vi "EnqueueMessage.vi"(8 "error in (no error)":errorcluster, 9 "Priority":u8, 10 "message":variant, 11 "queue in":refnum<data-value>) -> (0 "error out":errorcluster, 3 "queue out":refnum<data-value>)   [LabVIEW 2009, in "PriorityQueue.lvlib"]
uses:
  PriorityQueue.lvlib
  PriorityQueue/PriorityQueue.lvclass
  LLNode/LLNode.lvclass
  LinkedList/InsertSearch.ctl
  LLSearch/LLSearch.lvclass
  SearchPriority/SearchPriority.lvclass
  PriorityNode/PriorityNode.lvclass
  LinkedList/position.ctl
  LinkedList/LinkedList.lvclass
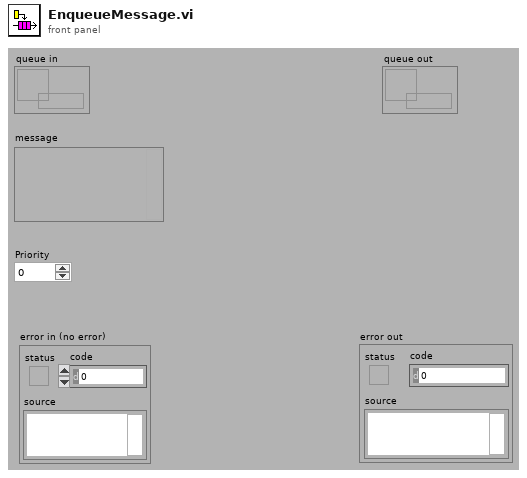
[diagram p1: front panel]
types:
  T1 = typedef "LinkedList.lvclass/InsertSearch.ctl" = cluster{"LLSearch in":refnum<class "LLSearch.lvclass">, "InsertIfEmpty":bool, "Insert After":bool, "InsertIfNotFound":bool}
  T2 = typedef "LinkedList.lvclass/position.ctl" = enum16{"Front", "Back", "Search"}
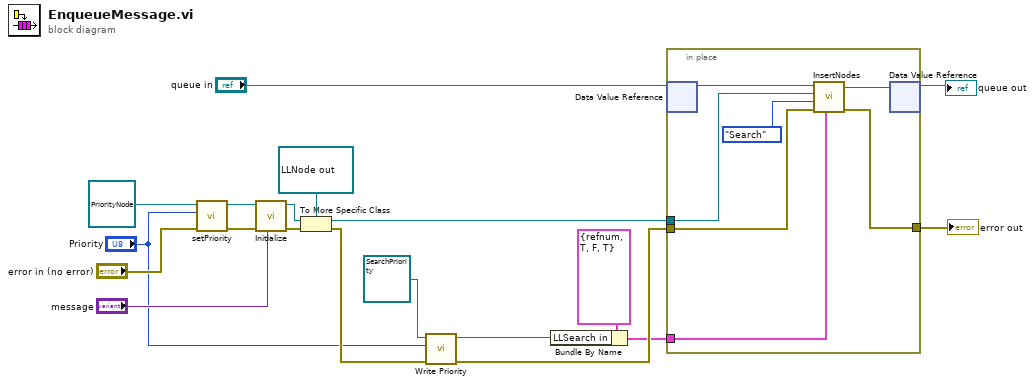
[diagram p0: block diagram]
diagram:
  n1 = call "setPriority.vi"("error in (no error)"="error in (no error)", "Priority"="Priority", "PriorityNode in"=refnum<class "PriorityNode.lvclass"> refnum ("PriorityNode.lvclass")) -> ("error out"=w2:errorcluster, "PriorityNode out"=w4:refnum<class "PriorityNode.lvclass">)  [unwired: 7 in]
  n2 = call-dynamic "Initialize.vi"("optional"="message", "error in (no error)"=w2, "PriorityNode data"=w4) -> ("error out"=w18:errorcluster, "Node out"=w17:refnum<data-value>)  [unwired: 7 in]
  n3 = To More Specific Class(target class=refnum<data-value> refnum ("ToInsert"), reference=w17, error in=w18) -> (specific class reference=w15:refnum<data-value>, error out=w13:errorcluster)
  n4 = call "Write Priority.vi"("error in (no error)"=w13, "Priority"="Priority", "SearchPriority in"=refnum<class "SearchPriority.lvclass"> refnum ("SearchPriority.lvclass")) -> ("error out"=w10:errorcluster, "SearchPriority out"=w11:refnum<class "SearchPriority.lvclass">)  [unwired: 7 in]
  n5 = Bundle By Name(cluster=T1 {"LLSearch in"=refnum, "InsertIfEmpty"=TRUE, "Insert After"=FALSE, "InsertIfNotFound"=TRUE} ("Insert Search"), "LLSearch in"=w11) -> (w9:T1)
  n6 = in-place {
    in-place-border: w15 -> [w22]
    in-place-border: w10 -> [w24]
    in-place-border: w9 -> [w23]
    in-place-border: [w20] -> w7
    n7 = in-place-dvr #1("queue in") -> (w26:refnum<class "PriorityQueue.lvclass">)  [unwired: 1 out]
    n8 = call "InsertNodes.vi"("Insert Search"=w23, "error in (no error)"=w24, "position"=position."Search", "ToInsert"=w22, "LinkedList in"=w26) -> ("error out"=w20:errorcluster, "LinkedList out"=w21:refnum<class "PriorityQueue.lvclass">)  [unwired: 4 in, 1 out]
    n9 = in-place-dvr #1(w21) -> (→"queue out":refnum<data-value>)  [unwired: 1 out]
  }
  "error out" <- w7
